vi "ImportBitmapTest.vi"() -> ()   [LabVIEW 2013, in "main.lvlib"]
uses:
  main.lvlib
  <vilib>/picture/picture.llb/imagedata.ctl
panel:
  in  "Test":bool
  in  "Close":bool
  out "status 2":bool
  out "status1":bool
  out "Metode 2":picture
  out "Metode 1":picture
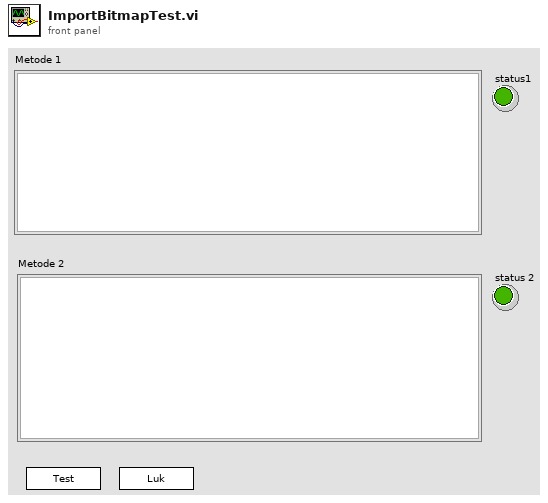
[diagram p1: front panel]
types:
  T1 = typedef "imagedata.ctl" = cluster{"image type":i32, "image depth":i32, "image":u8[], "mask":u8[], "colors":u32[], "Rectangle":cluster{"left":i16, "top":i16, "right":i16, "bottom":i16}}
  T2 = cluster{"left":i32, "top":i32, "right":i32, "bottom":i32}
  T3 = cluster{"left":i16, "top":i16, "right":i16, "bottom":i16}
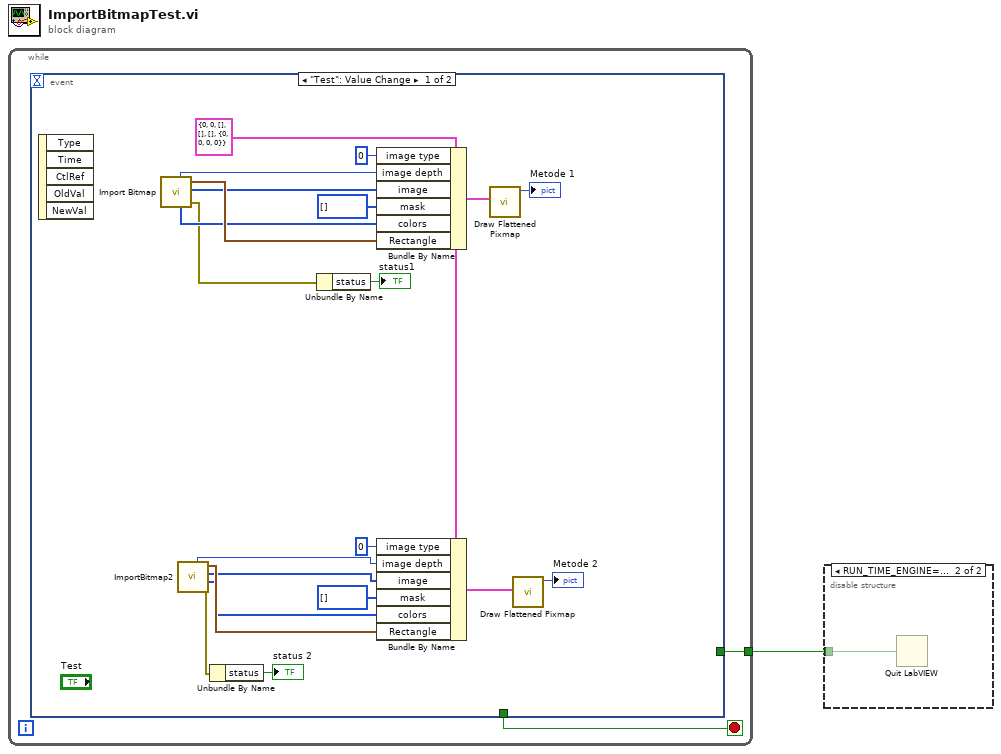
[diagram p0: block diagram]
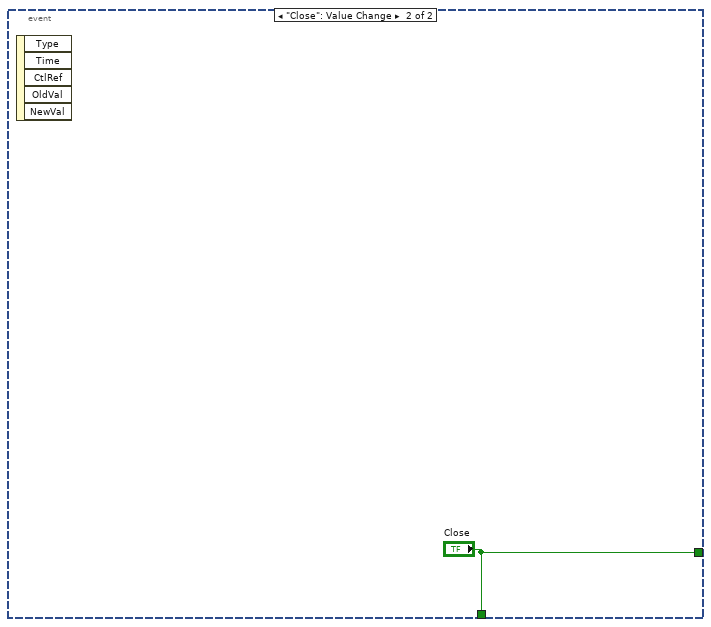
[diagram p3: hidden frame]
diagram:
  n1 = while {
    tunnel: [w2] -> w1
    stop <- w3 stop-if-true
    n2 = event shown="[0] \"Test\": Value Change" {
      selector: _ -> [_ _]
      dyn-events: _ -> [_ _]
      timeout: _ -> [_ _]
      tunnel: [_ "Close"] -> w3
      tunnel: [_ "Close"] -> w2
      event "Test": Value Change {
        w17 = T1 {"image type"=0, "image depth"=0, "image"=[], "mask"=[], "colors"=[], "Rectangle"={"left"=0, "top"=0, "right"=0, "bottom"=0}} ("image data")
        n3 = event-data() -> ()  [unwired: 1 in, 5 out]
        n4 = call "Import Bitmap.vi"() -> ("color depth"=w23:u8, "rect"=w22:T2, "flattened data"=w21:u8[], "color table"=w20:u32[], "error out"=w6:errorcluster)  [unwired: 5 in]
        n5 = call "ImportBitmap2.vi"() -> ("error out"=w7:errorcluster, "color table"=w15:u32[], "pixmap data"=w13:u8[], "rect"=w16:T3, "bit depth(8)"=w12:i32)  [unwired: 7 in]
        n6 = Unbundle By Name(w7) -> ("status"=→"status 2":bool)
        n7 = Unbundle By Name(w6) -> ("status"=→"status1":bool)
        n8 = Bundle By Name(cluster=w17, "image type"=0, "image depth"=w23, "image"=w21, "mask"=u8[] [], "colors"=w20, "Rectangle"=w22) -> (w18:T1)
        n9 = Bundle By Name(cluster=w17, "image type"=0, "image depth"=w12, "image"=w13, "mask"=u8[] [], "colors"=w15, "Rectangle"=w16) -> (w10:T1)
        n10 = call <vilib>:"Draw Flattened Pixmap.vi"("image data"=w18) -> ("new picture"=→"Metode 1":picture)  [unwired: 8 in]
        n11 = call <vilib>:"Draw Flattened Pixmap.vi"("image data"=w10) -> ("new picture"=→"Metode 2":picture)  [unwired: 8 in]
      }
      event "Close": Value Change {
        n12 = event-data() -> ()  [unwired: 1 in, 5 out]
      }
    }
  }
  n13 = disable-structure shown="RUN_TIME_ENGINE==True" {
    disable-tunnel: w1 -> [_ w26]
    frame condition #0 (active) {
    }
    frame condition #1 {
      n14 = Quit LabVIEW(quit? (T)=w26) -> ()
    }
  }
